vi "getLabelObj.vi"(8 "error in (no error)":errorcluster, 11 "Wire in":refnum<class "Wire.lvclass">) -> (0 "error out":errorcluster, 2 "label":refnum<class "TextDecoration.lvclass">, 3 "Wire out":refnum<class "Wire.lvclass">)   [LabVIEW 2023, in "TLC_Scripto.lvlib" / "Wire.lvclass"]
uses:
  Wire.lvclass
  TextDecoration/TextDecoration.lvclass
  Read wireRef.vi
  Wire.lvclass/Wire.ctl
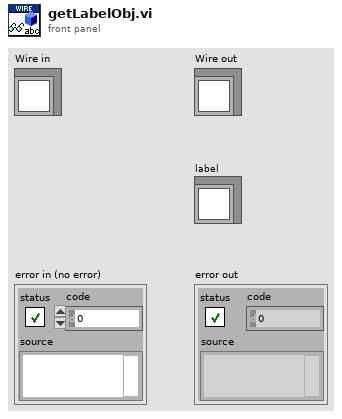
[diagram p1: front panel]
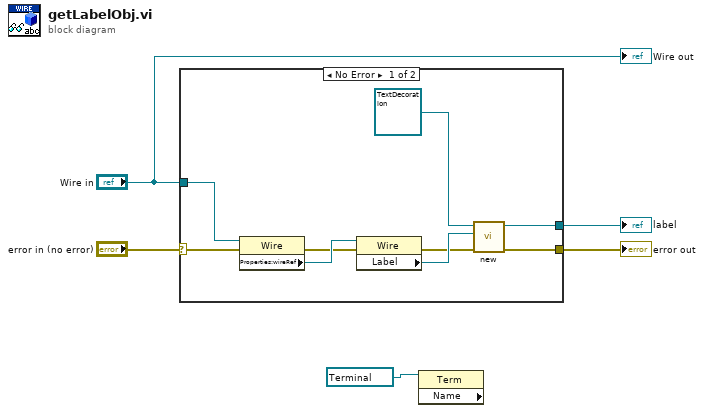
[diagram p0: block diagram]
diagram:
  n1 = case shown="No Error" "error in (no error)" {
    selector: "error in (no error)" -> [w12 w15]
    tunnel: "Wire in" -> [w14 _]
    tunnel: [w6 w15] -> w3
    tunnel: [w8 _] -> w2
    frame No Error {
      n2 = property class="Wire"(reference=w14, error in=w12) -> (error out=w11:errorcluster, "Properties:wireRef"=w13:refnum<vi>)  [unwired: 1 out]
      n3 = property class="Wire"(reference=w13, error in=w11) -> (error out=w7:errorcluster, "Label"=w9:refnum<vi>)  [unwired: 1 out]
      n4 = call-dynamic "new.vi"("Error In"=w7, "ref"=w9, "GObject in"=refnum<class "TextDecoration.lvclass"> refnum ("TLC_Scripto.lvlib:TextDecoration")) -> ("Error Out"=w6:errorcluster, "GObject out"=w8:refnum<class "TextDecoration.lvclass">)  [unwired: 7 in]
    }
    frame Error {
    }
  }
  "error out" <- w3
  "label" <- w2
  n5 = property class="Term" props=["Name"](reference=refnum<vi> refnum ("wireRef")) -> ()  [unwired: 1 in, 3 out]
  "Wire out" <- "Wire in"
